vi "UID Already Exists--error.vi"() -> (2 "Error":errorcluster)   [LabVIEW 2020, in "jettl.lvlib"]
uses:
  jettl.lvlib
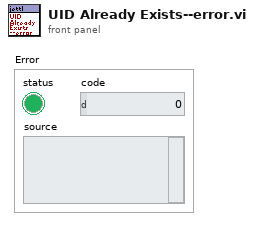
[diagram p1: front panel]
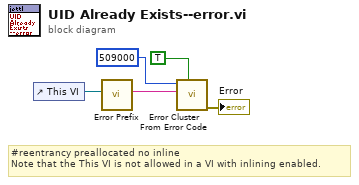
[diagram p0: block diagram]
diagram:
  # "#reentrancy preallocated no inline\nNote that the This VI is not allowed in a VI with inlining enabled."
  n1 = control-ref of="This VI"() -> (w2:refnum<vi>)
  n2 = call "Error Prefix.vi"("VI Ref"=w2) -> ("Prefix"=w1:string)  [unwired: 10 in]
  n3 = call <vilib>:"Error Cluster From Error Code.vi"("show call chain? (False)"=TRUE, "error message (\"\")"=w1, "error code (0)"=509000) -> ("error out"=→"Error":errorcluster)  [unwired: 6 in]
